vi "Robot_Recorder.vi"() -> ()   [LabVIEW 2016]
doc: "This VI implements the framework and scheduler for your robotics program. It should not be necessary to modify the framework. You are expected to add your code to the VIs called from Robot Main - the ones located in the Team Code folder within the project."
uses:
  <vilib>/Rock Robotics/WPI/ThirdParty/CanMotor/TalonSRX/WPI_CANTalonSRX_APIFeedbackSelect.ctl
  <vilib>/Rock Robotics/WPI/ThirdParty/CanMotor/TalonSRX/WPI_CANTalonSRX_APIControlMode.ctl
  <vilib>/Rock Robotics/WPI/ThirdParty/CanMotor/TalonSRX/WPI_CANTalonSRX_BrakeOverride.ctl
  <vilib>/Utility/file.llb/Write Delimited Spreadsheet (DBL).vi
panel:
  out "Revolutions":dbl
  out "Velocity - Right":dbl[](graph)
  out "Position - Right":dbl[](graph)
  out "Right Points":dbl[][](array[numeric])
  in  "OK Button":bool
  out "Position - Left":dbl[](graph)
  out "Velocity - Left":dbl[](graph)
  out "Left Points":dbl[][](array[numeric])
  in  "Stop":bool
  in  "Start":bool
  in  "?":bool
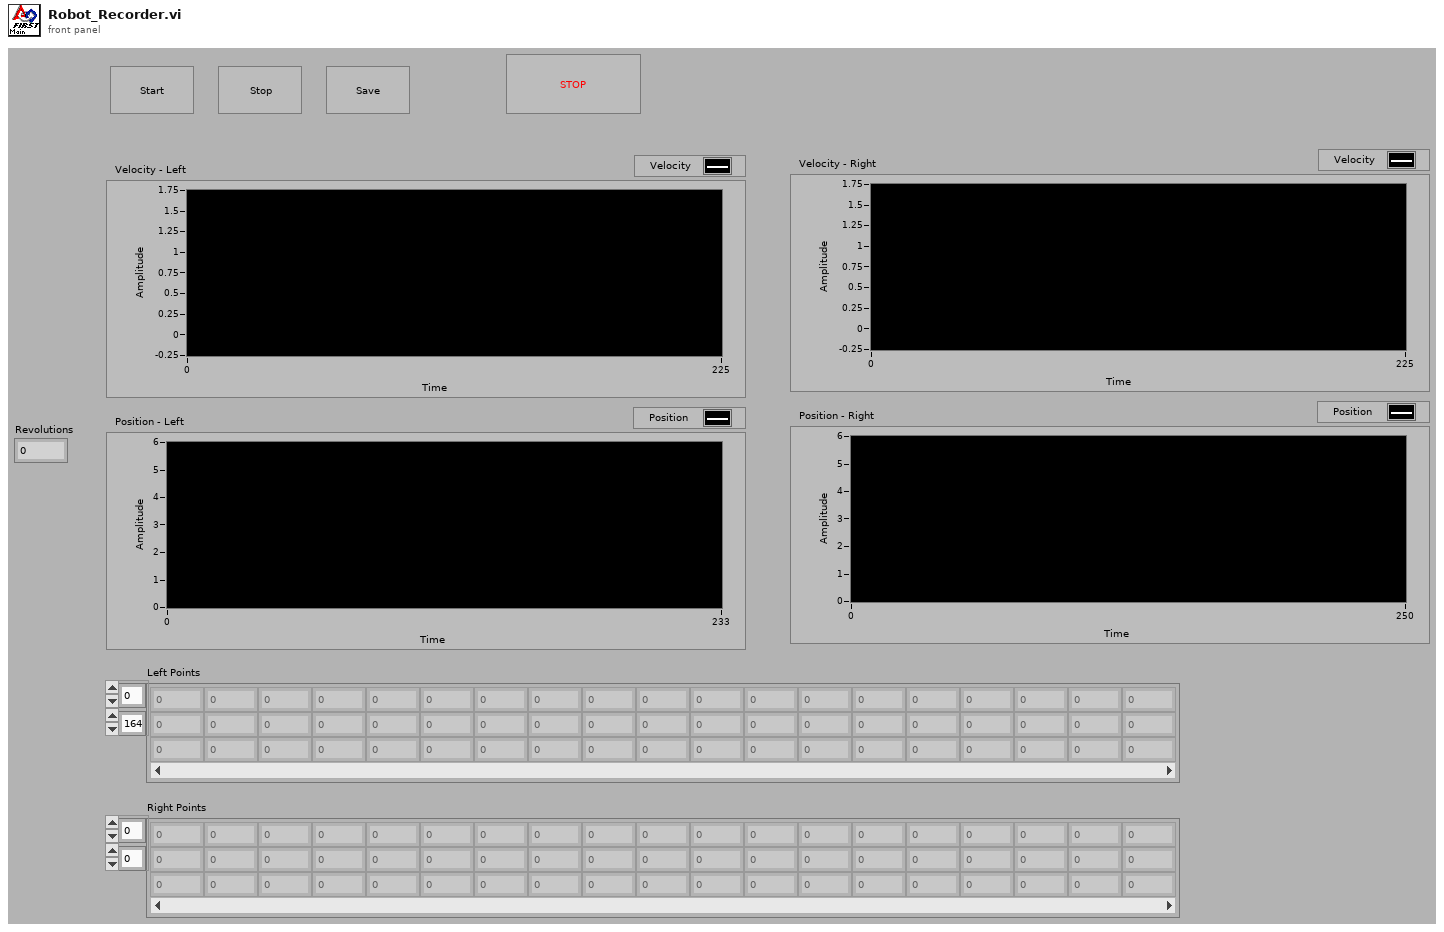
[diagram p1: front panel]
types:
  T1 = typedef "WPI_CANTalonSRX_APIFeedbackSelect.ctl" = enum16{"Digital Quadrature Encoder", "Analog Potentiometer", "Analog Encoder", "Count on Quad-A (Rising-Edge)", "Count on Quad-A (Falling-Edge)", "CTR Magnetic Enc (Absolute)", "CTR Magnetic Enc (Relative)", "Pulse Width"}
  T2 = typedef "WPI_CANTalonSRX_BrakeOverride.ctl" = enum8{"No Override", "Override to Coast", "Override to Brake"}
  T3 = typedef "WPI_CANTalonSRX_APIControlMode.ctl" = enum8{"Percent VBus", "Speed", "Position", "Slave", "Unchanged / Invalid", "Voltage Compensation", "Current", "Motion Profile", "Motion Magic"}
  T4 = typedef "WPI_MotorControlDeviceRef.ctl" = cluster{"DeviceStatus":errorcluster, "Type":T5, "PWM":cluster{"PWM Channel":T6, "DeadBand":T7}, "CAN":cluster{"Device Number":u8, "SetOutput VI Ref":variant, "GetOutput VI Ref":variant, "Enable VI Ref":variant, "Disable VI Ref":variant, "Data":variant}, "Invert":bool}
  T5 = typedef "WPI_MotorControlType.ctl" = enum16{"PWM", "CAN"}
  T6 = typedef "FPGA_DIOPWMChannel.ctl" = enum8{"PWM 0", "PWM 1", "PWM 2", "PWM 3", "PWM 4", "PWM 5", "PWM 6", "PWM 7", "PWM 8", "PWM 9", "PWM MXP 0", "PWM MXP 1", "PWM MXP 2", "PWM MXP 3", "PWM MXP 4", "PWM MXP 5", "PWM MXP 6", "PWM MXP 7", "PWM MXP 8", "PWM MXP 9", "Invalid"}
  T7 = typedef "WPI_PWMDeadband.ctl" = cluster{"Name":string, "maxPositivePwm":i32, "minPositivePwm":i32, "centerPwm":i32, "maxNegativePwm":i32, "minNegativePwm":i32, "angularRange":u16}
  T8 = typedef "WPI_CANTalonSRX_GlobalStatus.ctl" = cluster{"Applied Throttle":dbl, "Module Enabled":bool, "CAN Error":errorcluster, "Closed Loop Error":dbl, "Forward Limit Switch Closed":bool, "Reverse Limit Switch Closed":bool, "Sensor Position":dbl, "Sensor Velocity":dbl, "Current":dbl, "Sticky Fault - Over Temp":bool, "Sticky Fault - Under Voltage":bool, "Sticky Fault - Forward Limit":bool, "Sticky Fault - Reverse Limit":bool, "Sticky Fault - Forward Soft Limit":bool, "Sticky Fault - Reverse Soft Limit":bool, "Brake is Enabled":bool, "Encoder Position":dbl, "Encoder Velocity":dbl, "Encoder Index Count":dbl, "Encoder A Pin State":bool, "Encoder B Pin State":bool, "Encoder Index Pin State":bool, "Analog In":dbl, "Analog In Velocity":dbl, "Temperature (C)":dbl, "Battery Voltage":dbl, "Control 5 Is Supported":bool, "Current Profile Slot Select":dbl, "Pos Div 8":bool, "Vel Div 4":bool, "Pulse Width Position":i32, "Pulse Width Velocity":i32, "Pulse Width Rise To Rise (us)":i32, "Pulse Width Rise To Fall (us)":i32, "Mot Prof Active Is Under Run":bool, "Mot Prof Active Has Under Run":bool, "Mot Prof Active Is Last":bool, "Mot Prof Active Velocity Only":bool, "Mot Prof Active Is Valid":bool, "Mot Prof Buffer Is Full":bool, "Mot Prof Active Profile Slot Select":i32, "Mot Prof NextID":i32, "Mot Prof Count":i32, "Mot Prof Active Velocity":dbl, "Mot Prof Active Position":dbl, "Mot Prof Output Enable":i32, "UsageFrame":u32, "Motion Magic Active Trajectory":cluster{"Velocity":dbl, "Position":dbl}}
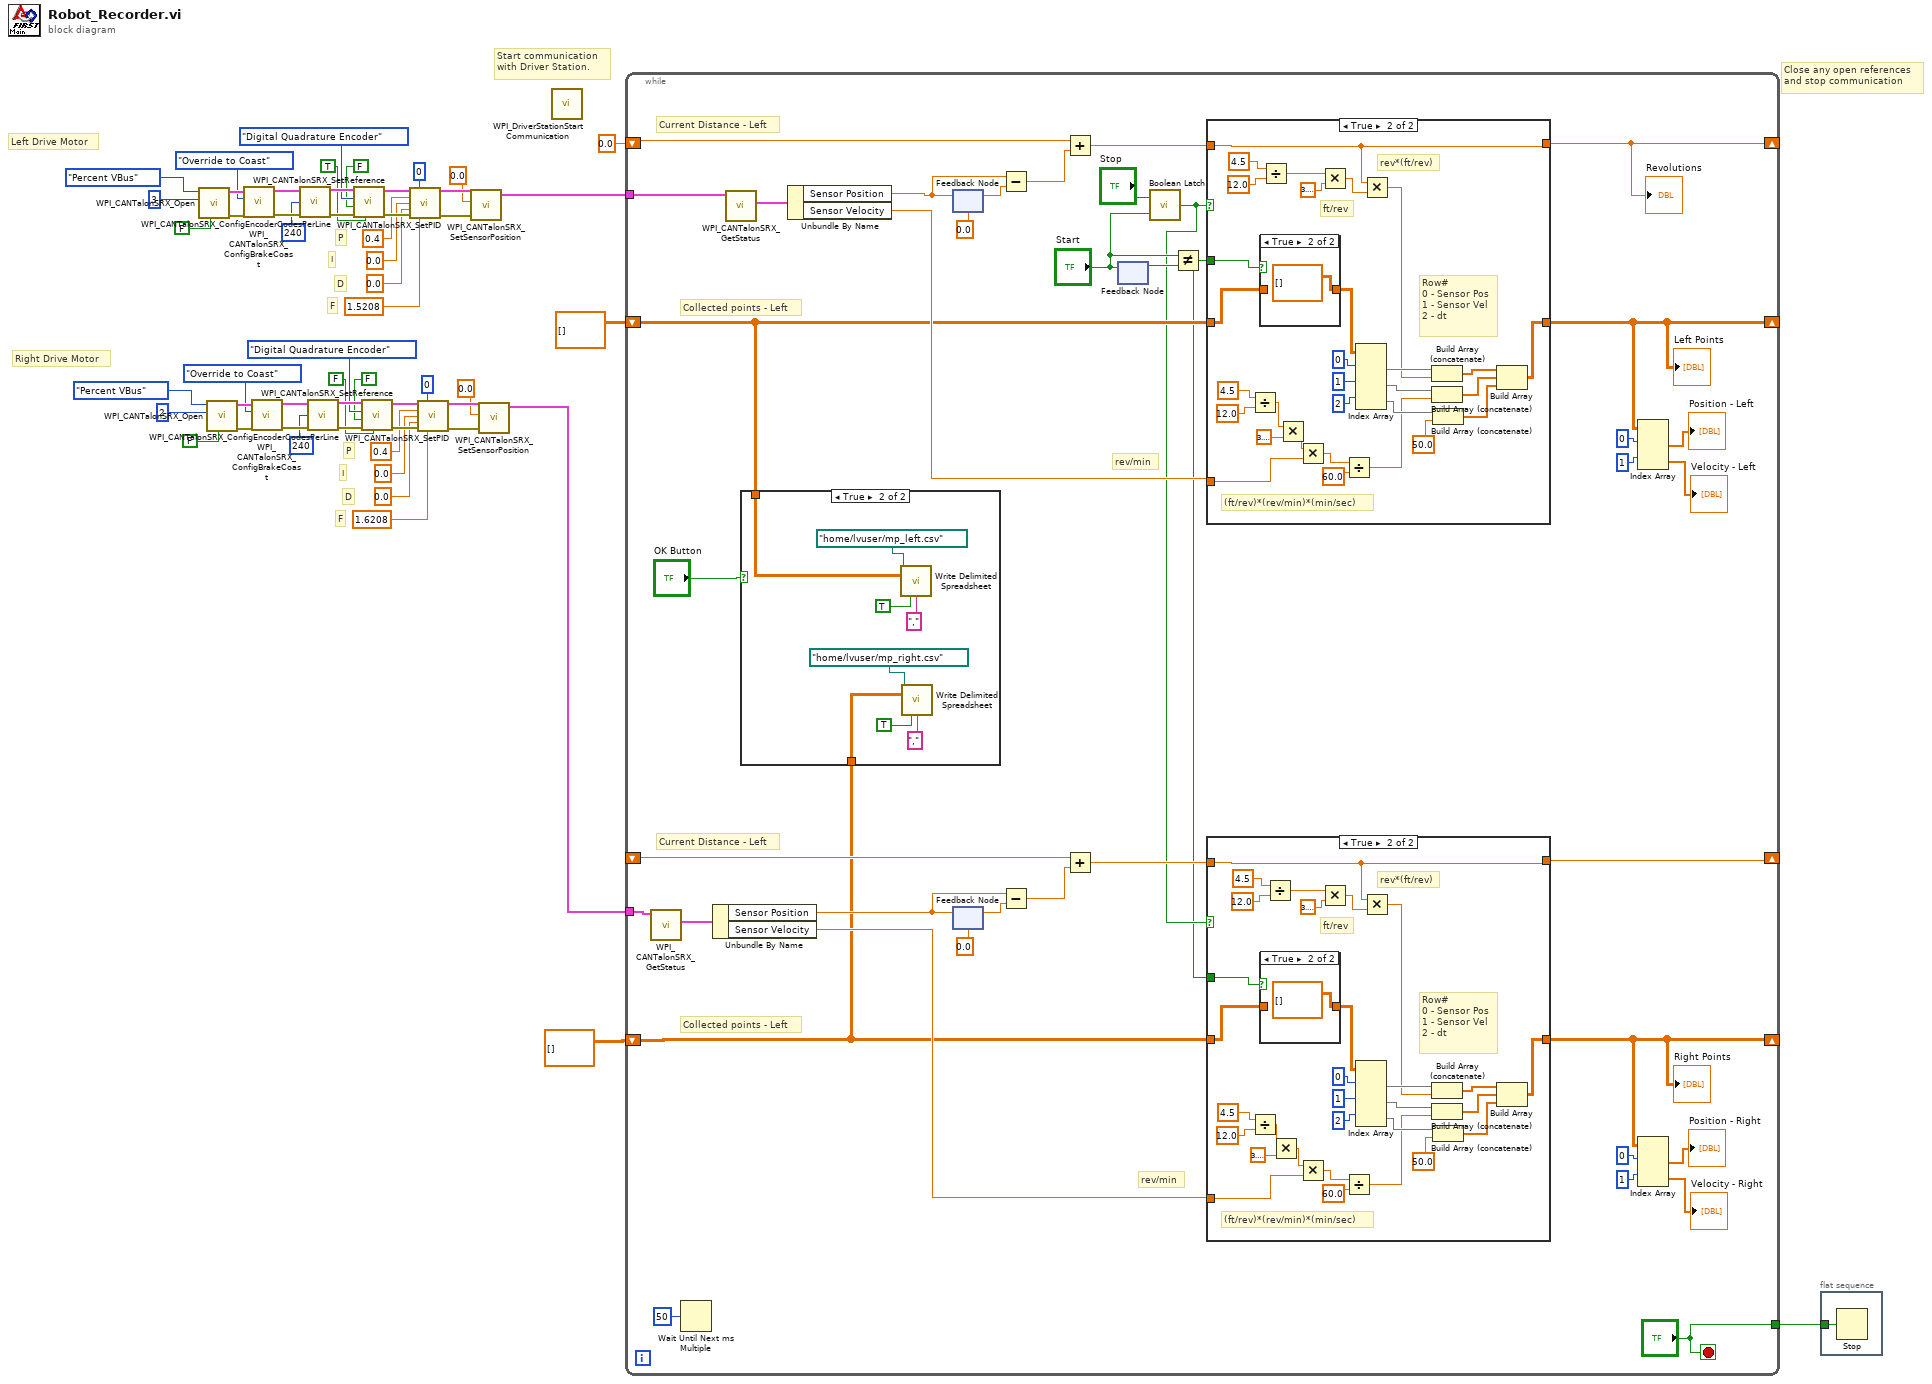
[diagram p0: block diagram]
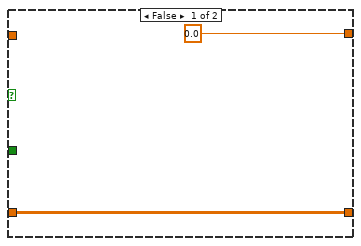
[diagram p2: hidden frame]
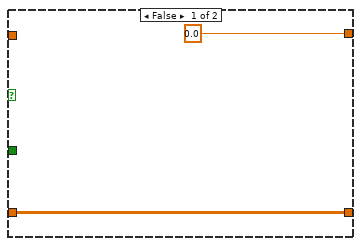
[diagram p5: hidden frame]
diagram:
  # "Right Drive Motor"
  # "Left Drive Motor"
  # "F"
  # "D"
  # "I"
  # "P"
  # "F"
  # "D"
  # "I"
  # "P"
  # "Close any open references\nand stop communication"
  # "Start communication\nwith Driver Station."
  n1 = call <vilib>:"WPI_CANTalonSRX_Open.vi"("Invert"=FALSE, "Device Number"=u8 3, "Control Mode"=WPI_CANTalonSRX_APIControlMode."Percent VBus") -> ("error out"=w51:errorcluster, "CAN Talon SRX Ref"=w50:T4)  [unwired: 7 in]
  n2 = call <vilib>:"WPI_CANTalonSRX_Open.vi"("Invert"=FALSE, "Device Number"=u8 2, "Control Mode"=WPI_CANTalonSRX_APIControlMode."Percent VBus") -> ("error out"=w27:errorcluster, "CAN Talon SRX Ref"=w26:T4)  [unwired: 7 in]
  n3 = call <vilib>:"WPI_CANTalonSRX_ConfigBrakeCoast.vi"("error in (no error)"=w51, "Brake / Coast Mode"=WPI_CANTalonSRX_BrakeOverride."Override to Coast", "CAN Talon SRX Ref"=w50) -> ("error out"=w47:errorcluster, "CAN Talon SRX Ref"=w48:T4)  [unwired: 7 in]
  n4 = call <vilib>:"WPI_CANTalonSRX_ConfigBrakeCoast.vi"("error in (no error)"=w27, "Brake / Coast Mode"=WPI_CANTalonSRX_BrakeOverride."Override to Coast", "CAN Talon SRX Ref"=w26) -> ("error out"=w23:errorcluster, "CAN Talon SRX Ref"=w24:T4)  [unwired: 7 in]
  n5 = call <vilib>:"WPI_CANTalonSRX_ConfigEncoderCodesPerLine.vi"("CAN Talon SRX Ref"=w48, "Number Encoder Lines\n(Counts Per Rotation)"=u32 240 ("Number Encoder Lines\n(Counts Per Rotation)"), "error in (no error)"=w47) -> ("CAN Talon SRX Ref"=w45:T4, "error out"=w43:errorcluster)  [unwired: 11 in]
  n6 = call <vilib>:"WPI_CANTalonSRX_ConfigEncoderCodesPerLine.vi"("CAN Talon SRX Ref"=w24, "Number Encoder Lines\n(Counts Per Rotation)"=u32 240 ("Number Encoder Lines\n(Counts Per Rotation)"), "error in (no error)"=w23) -> ("CAN Talon SRX Ref"=w21:T4, "error out"=w19:errorcluster)  [unwired: 11 in]
  n7 = call <vilib>:"WPI_CANTalonSRX_SetReference.vi"("Reverse Closed-Loop Output"=TRUE, "error in (no error)"=w43, "Reverse Feedback Sensor"=FALSE, "Feedback Reference"=WPI_CANTalonSRX_APIFeedbackSelect."Digital Quadrature Encoder", "CAN Talon SRX Ref"=w45) -> ("error out"=w41:errorcluster, "CAN Talon SRX Ref"=w42:T4)  [unwired: 5 in]
  n8 = call <vilib>:"WPI_CANTalonSRX_SetReference.vi"("Reverse Closed-Loop Output"=FALSE, "error in (no error)"=w19, "Reverse Feedback Sensor"=FALSE, "Feedback Reference"=WPI_CANTalonSRX_APIFeedbackSelect."Digital Quadrature Encoder", "CAN Talon SRX Ref"=w21) -> ("error out"=w17:errorcluster, "CAN Talon SRX Ref"=w18:T4)  [unwired: 5 in]
  n9 = call <vilib>:"WPI_CANTalonSRX_SetPID.vi"("CAN Talon SRX Ref"=w42, "Parameter Slot"=u8 0, "P"=0.4, "I"=0.0, "D"=0.0, "error in (no error)"=w41, "F"=1.5208) -> ("CAN Talon SRX Ref"=w33:T4, "error out"=w34:errorcluster)  [unwired: 7 in]
  n10 = call <vilib>:"WPI_CANTalonSRX_SetPID.vi"("CAN Talon SRX Ref"=w18, "Parameter Slot"=u8 0, "P"=0.4, "I"=0.0, "D"=0.0, "error in (no error)"=w17, "F"=1.6208) -> ("CAN Talon SRX Ref"=w9:T4, "error out"=w10:errorcluster)  [unwired: 7 in]
  n11 = call <vilib>:"WPI_CANTalonSRX_SetSensorPosition.vi"("error in (no error)"=w34, "New Sensor Position"=0.0, "CAN Talon SRX Ref"=w33) -> ("CAN Talon SRX Ref"=w5:T4)  [unwired: 7 in, 1 out]
  n12 = call <vilib>:"WPI_CANTalonSRX_SetSensorPosition.vi"("error in (no error)"=w10, "New Sensor Position"=0.0, "CAN Talon SRX Ref"=w9) -> ("CAN Talon SRX Ref"=w2:T4)  [unwired: 7 in, 1 out]
  n13 = call <vilib>:"WPI_DriverStationStart Communication.vi"() -> ()  [unwired: 2 in, 10 out]
  n14 = while {
    tunnel: ["?"] -> w54
    tunnel: w5 -> [w93]
    shift-right: [w87] -> _
    shift-left: 0.0 -> [w91]
    shift-right: [w79] -> _
    shift-left: dbl[][] [] -> [w73]
    shift-right: [w60] -> _
    shift-left: _ -> [w61]
    tunnel: w2 -> [w59]
    shift-right: [w58] -> _
    shift-left: dbl[][] [] -> [w57]
    stop <- "?" stop-if-true
    # "Collected points - Left"
    # "rev/min"
    # "Current Distance - Left"
    # "Collected points - Left"
    # "rev/min"
    # "Current Distance - Left"
    n15 = call <vilib>:"WPI_CANTalonSRX_GetStatus.vi"("CAN Talon SRX Ref"=w59) -> ("Talon SRX Status"=w72:T8)  [unwired: 8 in, 2 out]
    n16 = Wait Until Next ms Multiple(millisecond multiple=u32 50) -> ()  [unwired: 1 out]
    n17 = Unbundle By Name(w72) -> ("Sensor Position"=w67:dbl, "Sensor Velocity"=w66:dbl)
    n18 = call <vilib>:"WPI_CANTalonSRX_GetStatus.vi"("CAN Talon SRX Ref"=w93) -> ("Talon SRX Status"=w92:T8)  [unwired: 8 in, 2 out]
    n19 = case shown="True" "OK Button" {
      tunnel: w73 -> [_ w134]
      tunnel: w57 -> [_ w129]
      frame False {
      }
      frame True {
        n20 = call-poly <vilib>:"Write Delimited Spreadsheet.vi"("file path (dialog if empty)"=path "/home/lvuser/mp_left.csv" ("file path (use dialog)"), "2D data"=w134, "transpose? (no:F)"=TRUE, "delimiter (\\t)"="," ("delimiter (\\t)")) -> ()  [unwired: 10 in, 2 out]
        n21 = call-poly <vilib>:"Write Delimited Spreadsheet.vi"("file path (dialog if empty)"=path "/home/lvuser/mp_right.csv" ("file path (use dialog)"), "2D data"=w129, "transpose? (no:F)"=TRUE, "delimiter (\\t)"="," ("delimiter (\\t)")) -> ()  [unwired: 10 in, 2 out]
      }
    }
    n22 = Unbundle By Name(w92) -> ("Sensor Position"=w83:dbl, "Sensor Velocity"=w82:dbl)
    n23 = feedback-in #1(w83) -> ()
    n24 = feedback #1(0.0 ("Sensor Position")) -> (w90:dbl)
    n25 = feedback #2(0.0 ("Sensor Position")) -> (w71:dbl)
    n26 = feedback-in #2(w67) -> ()
    n27 = Subtract(x=w83, y=w90) -> (x-y=w89:dbl)
    n28 = Subtract(x=w67, y=w71) -> (x-y=w70:dbl)
    n29 = Add(x=w91, y=w89) -> (x+y=w88:dbl)
    n30 = Add(x=w61, y=w70) -> (x+y=w69:dbl)
    n31 = feedback-in #3("Start") -> ()
    n32 = feedback #3() -> (w81:bool)  [unwired: 1 in]
    n33 = call "Boolean Latch.vi"("Input"="Start", "Reset"="Stop") -> ("Output"=w56:bool)
    n34 = Not Equal?(x="Start", y=w81) -> (x != y?=w55:bool)
    n35 = case shown="True" w56 {
      tunnel: w88 -> [_ w151]
      tunnel: [0.0 w151] -> w87
      tunnel: w73 -> [w137 w167]
      tunnel: [w137 w165] -> w79
      tunnel: w82 -> [_ w147]
      tunnel: w55 -> [_ w168]
      frame False {
      }
      frame True {
        # "(ft/rev)*(rev/min)*(min/sec)"
        # "ft/rev"
        # "rev*(ft/rev)"
        # "Row#\n0 - Sensor Pos\n1 - Sensor Vel\n2 - dt"
        n36 = Divide(x=4.5, y=12.0) -> (x/y=w139:dbl)
        n37 = case shown="True" w168 {
          tunnel: [w169 dbl[][] []] -> w164
          tunnel: w167 -> [w169 _]
          frame False {
          }
          frame True {
          }
        }
        n38 = Divide(x=4.5, y=12.0) -> (x/y=w143:dbl)
        n39 = Multiply(x=w139, y=3.141592653589793) -> (x*y=w148:dbl)
        n40 = Multiply(x=w148, y=w147) -> (x*y=w146:dbl)
        n41 = Multiply(x=w143, y=3.141592653589793) -> (x*y=w152:dbl)
        n42 = Divide(x=w146, y=60.0) -> (x/y=w149:dbl)
        n43 = Index Array(array=w164, index (row) #1=0 ("index (row)"), index (row) #2=1 ("index (row)"), index (row) #3=2 ("index (row)")) -> (element #1=w160:dbl[], element #2=w159:dbl[], element #3=w158:dbl[])  [unwired: 3 in]
        n44 = Multiply(x=w151, y=w152) -> (x*y=w153:dbl)
        n45 = Build Array (concatenate)(w160, w153) -> (w166:dbl[])
        n46 = Build Array (concatenate)(w159, w149) -> (w156:dbl[])
        n47 = Build Array (concatenate)(w158, 50.0 ("element")) -> (w155:dbl[])
        n48 = Build Array(w166, w156, w155) -> (w165:dbl[][])
      }
    }
    "Left Points" <- w79
    "Revolutions" <- w87
    n49 = case shown="True" w56 {
      tunnel: w69 -> [_ w109]
      tunnel: [0.0 w109] -> w60
      tunnel: w57 -> [w95 w125]
      tunnel: [w95 w123] -> w58
      tunnel: w66 -> [_ w105]
      tunnel: w55 -> [_ w126]
      frame False {
      }
      frame True {
        # "(ft/rev)*(rev/min)*(min/sec)"
        # "ft/rev"
        # "rev*(ft/rev)"
        # "Row#\n0 - Sensor Pos\n1 - Sensor Vel\n2 - dt"
        n50 = Divide(x=4.5, y=12.0) -> (x/y=w97:dbl)
        n51 = case shown="True" w126 {
          tunnel: [w127 dbl[][] []] -> w122
          tunnel: w125 -> [w127 _]
          frame False {
          }
          frame True {
          }
        }
        n52 = Divide(x=4.5, y=12.0) -> (x/y=w103:dbl)
        n53 = Multiply(x=w97, y=3.141592653589793) -> (x*y=w106:dbl)
        n54 = Multiply(x=w106, y=w105) -> (x*y=w104:dbl)
        n55 = Multiply(x=w103, y=3.141592653589793) -> (x*y=w110:dbl)
        n56 = Divide(x=w104, y=60.0) -> (x/y=w107:dbl)
        n57 = Index Array(array=w122, index (row) #1=0 ("index (row)"), index (row) #2=1 ("index (row)"), index (row) #3=2 ("index (row)")) -> (element #1=w118:dbl[], element #2=w117:dbl[], element #3=w116:dbl[])  [unwired: 3 in]
        n58 = Multiply(x=w109, y=w110) -> (x*y=w111:dbl)
        n59 = Build Array (concatenate)(w118, w111) -> (w124:dbl[])
        n60 = Build Array (concatenate)(w117, w107) -> (w114:dbl[])
        n61 = Build Array (concatenate)(w116, 50.0 ("element")) -> (w113:dbl[])
        n62 = Build Array(w124, w114, w113) -> (w123:dbl[][])
      }
    }
    "Right Points" <- w58
    n63 = Index Array(array=w79, index (row) #1=0 ("index (row)"), index (row) #2=1 ("index (row)")) -> (element #1=→"Position - Left":dbl[], element #2=→"Velocity - Left":dbl[])  [unwired: 2 in]
    n64 = Index Array(array=w58, index (row) #1=0 ("index (row)"), index (row) #2=1 ("index (row)")) -> (element #1=→"Position - Right":dbl[], element #2=→"Velocity - Right":dbl[])  [unwired: 2 in]
  }
  n65 = flat-sequence {
    tunnel: w54 -> [w171]
    frame #0 {
      n66 = Stop(stop? (T)=w171) -> ()
    }
  }
